vi "3 state controller.vi"(9 "Power":dbl, 10 "Backward":bool, 11 "Forward":bool) -> (3 "Numeric":dbl)   [LabVIEW 2012]
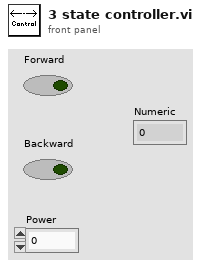
[diagram p1: front panel]
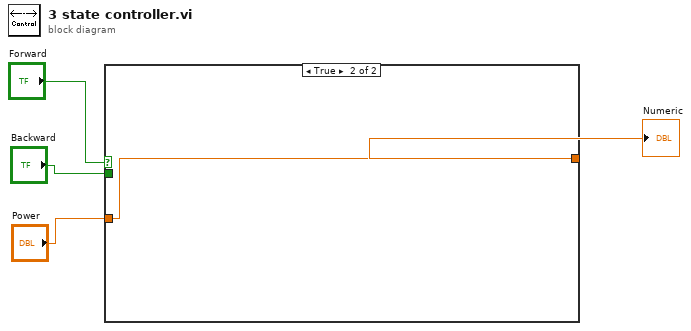
[diagram p0: block diagram]
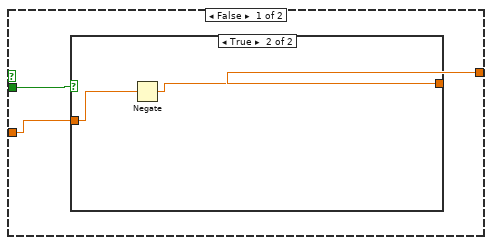
[diagram p2: hidden frame]
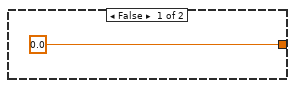
[diagram p3: hidden frame]
diagram:
  n1 = case shown="True" "Forward" {
    tunnel: "Power" -> [w6 w11]
    tunnel: [w5 w11] -> w2
    tunnel: "Backward" -> [w7 _]
    frame False {
      n2 = case shown="True" w7 {
        tunnel: w6 -> [_ w10]
        tunnel: [0.0 w9] -> w5
        frame False {
        }
        frame True {
          n3 = Negate(x=w10) -> (-x=w9:dbl)
        }
      }
    }
    frame True {
    }
  }
  "Numeric" <- w2
